vi "testNetworkCam.vi"() -> ()   [LabVIEW 2009, in "run.lvlib"]
uses:
  run.lvlib
  Tools/Filing/FileSystem/FileSystem.lvclass
  Tools/CameraSettings/CamaraSettings.lvclass
  HWController/Network Controllers/NetworkCamera/NetworkCamera.lvclass
  Tools/Filing/FileNeologist/FileNeologist.lvclass
panel:
  in  "stop 2":bool
  out "stopped 2":bool
  in  "run image viewer":bool
  in  "stop":bool
  out "stopped":bool
  in  "number":i32=-1
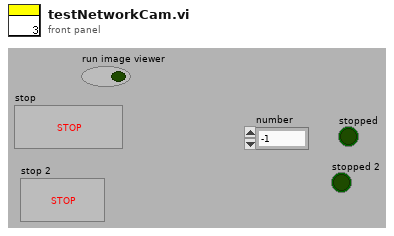
[diagram p1: front panel]
types:
  T1 = enum32{"Invalid", "Standard", "Closed", "Hidden", "Minimized", "Maximized"}
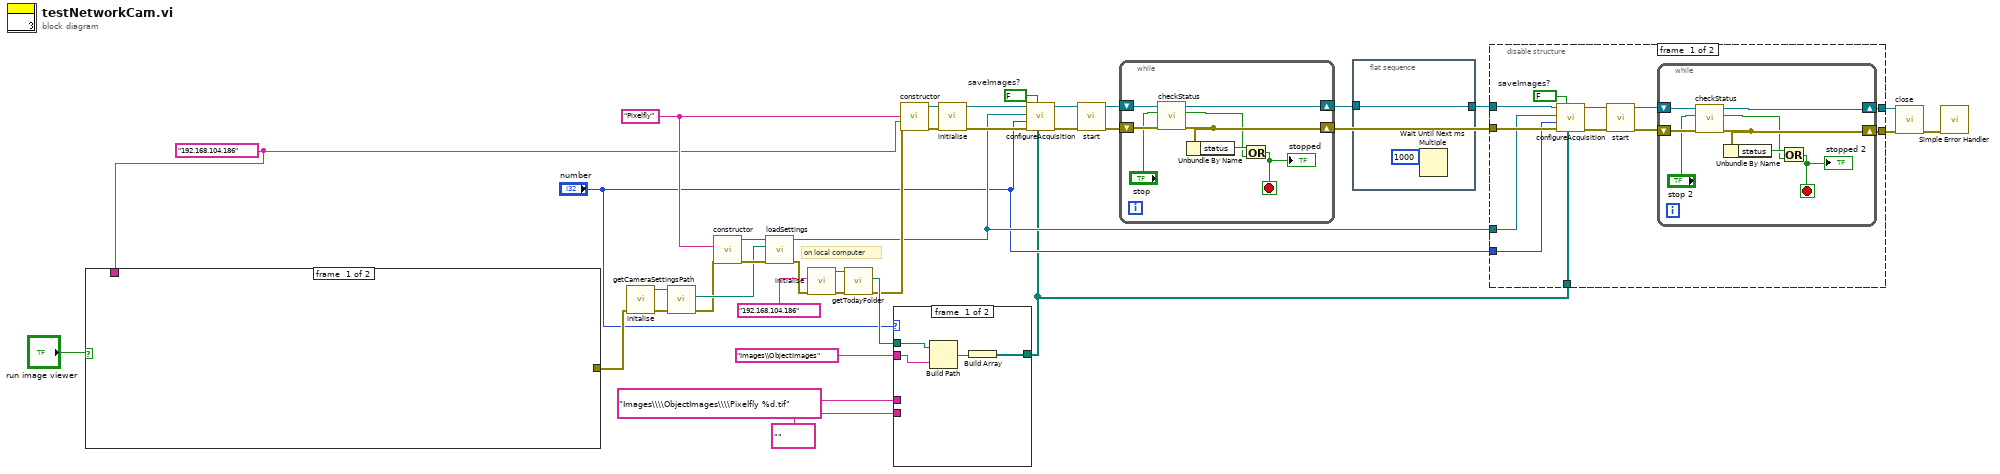
[diagram p0: block diagram]
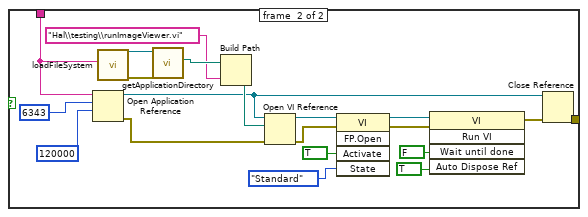
[diagram p3: hidden frame]
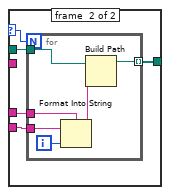
[diagram p4: hidden frame]
diagram:
  w19 = FALSE  # saveImages?
  w11 = "192.168.104.186"
  w16 = "Pixelfly"
  # "on local computer"
  n1 = case shown="True" "run image viewer" {
    tunnel: w11 -> [_ w57]
    tunnel: [_ w56] -> w10
    frame #0 {
    }
    frame #1 {
      n2 = Open Application Reference(9:120000 ("timeout ms (60000)"), 10:u16 6343 ("port number or service name (3363)"), 11:w57) -> (0:w55:errorcluster, 3:w46:refnum<vi>)  [unwired: 1 in]
      n3 = call "loadFileSystem.vi"("computer name"=w57) -> ("error out"=w53:errorcluster, "FileSystem out"=w54:refnum<class "FileSystem.lvclass">)  [unwired: 9 in]
      n4 = call-dynamic "getApplicationDirectory.vi"("error in (no error)"=w53, "FileSystem.lvclass in"=w54) -> ("ApplicationDirectory"=w52:path)  [unwired: 7 in, 2 out]
      n5 = Build Path(base path=w52, name or relative path="Hal\\testing\\runImageViewer.vi") -> (appended path=w50:path)
      n6 = Open VI Reference(application reference (local)=w46, vi path=w50, error in (no error)=w55) -> (vi reference=w49:refnum<vi>, error out=w40:errorcluster)  [unwired: 3 in]
      n7 = invoke class="VI" method="FP.Open"(reference=w49, error in=w40, "Activate"=TRUE ("Activate?"), "State"=T1."Standard") -> (reference out=w43:refnum<vi>, error out=w39:errorcluster)  [unwired: 1 in, 3 out]
      n8 = invoke class="VI" method="Run VI"(reference=w43, error in=w39, "Wait until done"=FALSE, "Auto Dispose Ref"=TRUE ("Auto Dispose Reference")) -> (error out=w45:errorcluster)  [unwired: 1 in, 4 out]
      n9 = Close Reference(reference=w46, error in (no error)=w45) -> (error out=w56:errorcluster)
    }
  }
  n10 = call "initalise.vi"("error in (no error)"=w10) -> ("error out"=w32:errorcluster, "FileSystem out"=w33:refnum<class "FileSystem.lvclass">)  [unwired: 9 in]
  n11 = call-dynamic "getCameraSettingsPath.vi"("error in (no error)"=w32, "FileSystem.lvclass in"=w33) -> ("error out"=w30:errorcluster, "CameraSettingsPath"=w31:path)  [unwired: 7 in, 1 out]
  n12 = call "constructor.vi"("error in (no error)"=w30, "camera settings"=w16) -> ("error out"=w34:errorcluster, "CamaraSettings out"=w35:refnum<class "CamaraSettings.lvclass">)  [unwired: 8 in]
  n13 = call-dynamic "loadSettings.vi"("error in (no error)"=w34, "Path"=w31, "CamaraSettings in"=w35) -> ("error out"=w29:errorcluster, "CamaraSettings out"=w7:refnum<class "CamaraSettings.lvclass">)  [unwired: 7 in]
  n14 = call "initialise.vi"("error in (no error)"=w29, "computer name"="192.168.104.186") -> ("error out"=w27:errorcluster, "FileNeologist out"=w28:refnum<class "FileNeologist.lvclass">)  [unwired: 8 in]
  n15 = call "getTodayFolder.vi"("error in (no error)"=w27, "FileNeologist in"=w28) -> ("error out"=w20:errorcluster, "todayFolder"=w26:path)  [unwired: 7 in, 1 out]
  n16 = case shown="1, Default" "number" {
    selector: "number" -> [_ w63]
    tunnel: w26 -> [w60 w66]
    tunnel: [w61 w65] -> w5
    tunnel: "Images\\\\ObjectImages\\\\Pixelfly %d.tif" -> [_ w64]
    tunnel: "" -> [_ w62]
    tunnel: "Images\\ObjectImages" -> [w59 _]
    frame #0 {
      n17 = Build Path(base path=w60, name or relative path=w59) -> (appended path=w58:path)
      n18 = Build Array(w58) -> (w61:path[])
    }
    frame #1 {
      n19 = for {
        N: w63 -> [_]
        tunnel: w66 -> [w72]
        tunnel: [w71] -> w65 mode=indexing
        tunnel: w64 -> [w69]
        tunnel: w62 -> [w67]
        i -> [w70]
        n20 = Format Into String(format string=w69, initial string=w67, w70) -> (resulting string=w68:string)  [unwired: 1 in, 1 out]
        n21 = Build Path(base path=w72, name or relative path=w68) -> (appended path=w71:path)
      }
    }
  }
  n22 = call "constructor.vi"("error in (no error)"=w20, "machine name"=w11, "Camera"=w16) -> ("error out"=w36:errorcluster, "NetworkCamera out"=w37:refnum<class "NetworkCamera.lvclass">)  [unwired: 7 in]
  n23 = call-dynamic "initialise.vi"("error in (no error)"=w36, "NetworkCamera in"=w37) -> ("error out"=w21:errorcluster, "NetworkCamera out"=w22:refnum<class "NetworkCamera.lvclass">)  [unwired: 8 in]
  n24 = call-dynamic "configureAcquisition.vi"("imagePaths"=w5, "saveImages?"=w19, "error in (no error)"=w21, "number of Images"="number", "CamaraSettings"=w7, "NetworkCamera in"=w22) -> ("error out"=w17:errorcluster, "NetworkCamera out"=w18:refnum<class "NetworkCamera.lvclass">)  [unwired: 4 in]
  n25 = call-dynamic "start.vi"("error in (no error)"=w17, "NetworkCamera in"=w18) -> ("error out"=w14:errorcluster, "NetworkCamera out"=w15:refnum<class "NetworkCamera.lvclass">)  [unwired: 8 in]
  n26 = while {
    shift-right: [w77] -> w1
    shift-left: w15 -> [w78]
    shift-right: [w75] -> w8
    shift-left: w14 -> [w76]
    stop <- w79 stop-if-true
    n27 = call-dynamic "checkStatus.vi"("error in (no error)"=w76, "stop"="stop", "NetworkCamera in"=w78) -> ("error out"=w75:errorcluster, "stopped?"=w74:bool, "NetworkCamera out"=w77:refnum<class "NetworkCamera.lvclass">)  [unwired: 6 in]
    n28 = Unbundle By Name(w75) -> ("status"=w80:bool)
    n29 = Or(x=w80, y=w74) -> (x .or. y?=w79:bool)
    "stopped" <- w79
  }
  n30 = flat-sequence {
    tunnel: [w82] -> w2
    tunnel: w1 -> [w82]
    frame #0 {
      n31 = Wait Until Next ms Multiple(millisecond multiple=1000) -> ()  [unwired: 1 out]
    }
  }
  n32 = disable-structure shown="Enabled" {
    disable-tunnel: w8 -> [w94 w103]
    disable-tunnel: w7 -> [w93 _]
    disable-tunnel: "number" -> [w92 _]
    disable-tunnel: w5 -> [w91 _]
    disable-tunnel: [w90 w104] -> w4
    disable-tunnel: [w89 w103] -> w3
    disable-tunnel: w2 -> [w88 w104]
    frame #0 {
      w87 = FALSE  # saveImages?
      n33 = call-dynamic "configureAcquisition.vi"("imagePaths"=w91, "saveImages?"=w87, "error in (no error)"=w94, "number of Images"=w92, "CamaraSettings"=w93, "NetworkCamera in"=w88) -> ("error out"=w85:errorcluster, "NetworkCamera out"=w86:refnum<class "NetworkCamera.lvclass">)  [unwired: 4 in]
      n34 = call-dynamic "start.vi"("error in (no error)"=w85, "NetworkCamera in"=w86) -> ("error out"=w83:errorcluster, "NetworkCamera out"=w84:refnum<class "NetworkCamera.lvclass">)  [unwired: 8 in]
      n35 = while {
        shift-right: [w99] -> w90
        shift-left: w84 -> [w100]
        shift-right: [w97] -> w89
        shift-left: w83 -> [w98]
        stop <- w101 stop-if-true
        n36 = call-dynamic "checkStatus.vi"("error in (no error)"=w98, "stop"="stop 2", "NetworkCamera in"=w100) -> ("error out"=w97:errorcluster, "stopped?"=w96:bool, "NetworkCamera out"=w99:refnum<class "NetworkCamera.lvclass">)  [unwired: 6 in]
        n37 = Unbundle By Name(w97) -> ("status"=w102:bool)
        n38 = Or(x=w102, y=w96) -> (x .or. y?=w101:bool)
        "stopped 2" <- w101
      }
    }
    frame #1 {
    }
  }
  n39 = call-dynamic "close.vi"("error in (no error)"=w3, "NetworkCamera in"=w4) -> ("error out"=w13:errorcluster)  [unwired: 9 in]
  n40 = call <vilib>:"Simple Error Handler.vi"("error in (no error)"=w13) -> ()  [unwired: 4 in, 5 out]
